vi "Stop Core.vi"(10 "final error code":i32, 11 "RPI.SenseHat.Actor in":refnum<class "RPI.SenseHat.Actor.lvclass">) -> (3 "RPI.SenseHat.Actor out":refnum<class "RPI.SenseHat.Actor.lvclass">)   [LabVIEW 2020, in "RPI.SenseHat.Actor.lvlib" / "RPI.SenseHat.Actor.lvclass"]
doc: "(<B>Filename</B>: Actor Framework.lvlib:Actor.lvclass:Stop Core.vi)\n\nDefines what the actor does before it stops. Use the <B>final error code</B> input to determine whether the actor shut down in response to an error.\n\nBy default, this method passes the Stop message along to all auto-stop nested actors. A descendant class may override this method to define additional behavior, such as shutting down any processes the actor initiated in its override of the Actor Core method."
uses:
  RPI.SenseHat.Actor.lvclass
  RPI.SenseHat.Actor.lvclass/RPI.SenseHat.Actor.ctl
  <vilib>/ActorFramework/Actor/Actor.lvclass
  RPI.SenseHat/SenseHat/SenseHat.lvclass
  <vilib>/MakerHub/LINX/LMH-LINX.lvlib
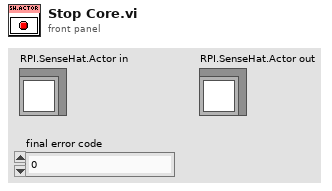
[diagram p1: front panel]
types:
  T1 = typedef "LMH-LINX.lvlib/LINX Ref.ctl" = cluster{"IO":T2, "Interface":T3, "LINX Device Config":T4}
  T2 = typedef "LMH-LINX.lvlib/Platform.ctl" = enum16{"Remote", "Local"}
  T3 = typedef "LMH-LINX.lvlib/Interface.ctl" = enum16{"Serial", "TCP"}
  T4 = typedef "LMH-LINX.lvlib/Device.lvlib/LINX Device Config.ctl" = cluster{"Interface":T3, "COM Port":refnum<visa-resource-name>, "TCP Configuration":T5, "Device Family":u8, "Device ID":u8, "Device Name":string, "TCP Ref":refnum<k5>, "Channels":T6}
  T5 = typedef "LMH-LINX.lvlib/Device.lvlib/TCP Config.ctl" = cluster{"IP Address":string, "Port":u16}
  T6 = typedef "LMH-LINX.lvlib/Channels.ctl" = cluster{"DI":u8[], "DO":u8[], "AI":u8[], "AO":u8[], "PWM":u8[], "QE":u8[], "UART":u8[], "I2C 2":u8[], "SPI":u8[], "CAN":u8[], "Servo":u8[], "AI Ref (V)":dbl, "AI Resolution (Bits)":u8, "AO Ref (V)":dbl, "AO Resolution (Bits)":u8}
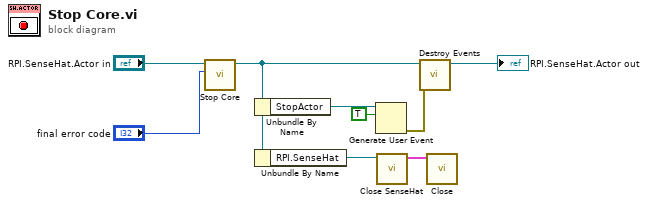
[diagram p0: block diagram]
diagram:
  n1 = call-parent "Stop Core.vi"("final error code"="final error code", "Actor in"="RPI.SenseHat.Actor in") -> ("Actor out"=w3:refnum<class "RPI.SenseHat.Actor.lvclass">)  [unwired: 9 in]
  n2 = Unbundle By Name(w3) -> ("StopActor"=w6:refnum<user-event>)
  n3 = Unbundle By Name(w3) -> ("RPI.SenseHat"=w2:refnum<class "SenseHat.lvclass">)
  n4 = Generate User Event(user event=w6, event data cluster=TRUE ("event data")) -> (error out=w4:errorcluster)  [unwired: 2 in, 1 out]
  n5 = call "Close SenseHat.vi"("SenseHat in"=w2) -> ("LINX Resource"=w1:T1)  [unwired: 9 in, 1 out]
  n6 = call "Destroy Events.vi"("error in (no error)"=w4, "RPI.SenseHat.Actor in"=w3) -> ("RPI.SenseHat.Actor out"=→"RPI.SenseHat.Actor out":refnum<class "RPI.SenseHat.Actor.lvclass">)  [unwired: 8 in, 1 out]
  n7 = call <vilib>:"Close.vi"("LINX Resource"=w1) -> ()  [unwired: 10 in, 1 out]
